vi "Select server and param_DO.vi"(0 "Activate":bool) -> (3 "This VI":refnum<vi>, 4 "host out":T1, 6 "HOST OK":bool, 12 "DI OK":bool, 13 "DI":string[](array[string]), 14 "DI table out":string="EP_XQ.1801" caption="таблица дискретных параметров")   [LabVIEW 2019]
uses:
  Database/PostgreSQL2LabVIEW/libpqlv/src/PQconnectdb.vi
  Database/PostgreSQL2LabVIEW/libpqlv/src/PQerrorMessage.vi
  Database/PostgreSQL2LabVIEW/libpqlv/src/PQstatus.vi
  Database/PostgreSQL2LabVIEW/libpqUtility/src/PQgetColumn.vi
  Database/PostgreSQL2LabVIEW/libpqUtility/src/PQclose.vi
  Database/select_initial.vi
  Database/PostgreSQL2LabVIEW/libpqlv/src/PQgetResult.vi
  Database/PostgreSQL2LabVIEW/libpqlv/src/PQclear.vi
  Database/PostgreSQL2LabVIEW/libpqUtility/src/PQfetchTables.vi
  Database/PostgreSQL2LabVIEW/libpqlv/src/PQresultErrorMessage.vi
  Database/PostgreSQL2LabVIEW/libpqlv/src/PQresultStatus.vi
  Database/PostgreSQL2LabVIEW/libpqlv/src/PQsendQuery.vi
  Database/PostgreSQL2LabVIEW/libpqlv/src/PQgetvalue.vi
  Database/PostgreSQL2LabVIEW/libpqlv/src/PQntuples.vi
  Database/PostgreSQL2LabVIEW/libpqUtility/src/PQgetTable.vi
  Database/Progress.vi
  Database/PostgreSQL2LabVIEW/libpqUtility/libpqutility.lvlib
  Database/PostgreSQL2LabVIEW/libpqlv/libpqlv.lvlib
  Inputs.lvlib
panel:
  in  "Param":i32[](listbox) caption="Параметры"
  in  "DI0":u16(ring) items=["EB31TB1_XB01", "EB31TB1_XB02", "EB31TB1_XB47", "EB321TB1_XB01", "EB321TB1_XB02", "EB321TB1_XB47", "EB322TB1_XB01", "EB322TB1_XB02", "EB322TB1_XB47", "EB323TB1_XB01", "EB323TB1_XB02", "EB323TB1_XB47", "EPCL1QM1_XB01", "EPCL1QM1_XB02", "EPCL1QM1_XB24", "EPG1GP1_XB01", "EPG1GP1_XB02", "EPG1GP1_XB19", "EPG1GP1_XB24", "EPG1GP2_XB01", "EPG1GP2_XB02", "EPG1GP2_XB19", "EPG1GP2_XB24", "EPG2GP1_XB01", "EPG2GP1_XB02", "EPG2GP1_XB19", "EPG2GP1_XB24", "EPG2GP2_XB01", "EPG2GP2_XB02", "EPG2GP2_XB19", "EPG2GP2_XB24", "EPG2GP3_XB01", "EPG2GP3_XB02", "EPG2GP3_XB19", "EPG2GP3_XB24", "EPG3GP1_XB01", "EPG3GP1_XB02", "EPG3GP1_XB19", "EPG3GP1_XB24", "EPG3GP2_XB01", "EPG3GP2_XB02", "EPG3GP2_XB19", "EPG3GP2_XB24", "EPHQ_XB01", "EPHQ_XB24", "EPKF1_A11", "EPKF1_A12", "EPKF1_A13", "EPKF1_A14", "EPKF1_A15", "EPKF2_A1", "EPKF2_A2", "EPKF2_A3", "GM31QM3_XB01", "GM31QM3_YB01", "GM31QM4_XB01", "GM31QM4_YB01", "HXQM1_XB01", "HXQM2_XB01", "HXQM3_XB01", "HXQM4_XB01", "HXQM5_XB01", "W1QM1_XB01", "W1QM1_YB01", "W1QM21_XB01", "W1QM21_YB01", "W1QM22_XB01", "W1QM22_YB01", "W1QM2_XB01", "W1QM2_YB01", "W1QM311_XB01", "W1QM311_YB01", "W1QM312_XB01", "W1QM312_YB01", "W1QM31_XB01", "W1QM31_YB01", "W1QM32_XB01", "W1QM32_YB01", "W1QM33_XB01", "W1QM33_YB01", "W1QM34_XB01", "W1QM34_YB01", "W1QM35_XB01", "W1QM35_YB01", "W1QM4_XB01", "W1QM4_YB01", "W1QM5_XB01", "W1QM5_YB01"]
  in  "DIParameters table":dbl[][](array[numeric])=[[0.0, 0.0, 3.0, 0.0], [0.0, 0.0, 3.0, 1.0], [0.0, 0.0, 0.0, 0.0], [0.0, 0.0, 3.0, 2.0], [0.0, 0.0, 3.0, 3.0], [0.0, 0.0, 3.0, 4.0], [0.0, 0.0, 0.0, 1.0], [0.0, 0.0, 3.0, 5.0], [0.0, 0.0, 4.0, 0.0], [0.0, 0.0, 4.0, 1.0], [0.0, 0.0, 0.0, 2.0], [0.0, 0.0, 4.0, 2.0], [0.0, 0.0, 4.0, 3.0], [0.0, 0.0, 4.0, 4.0], [0.0, 0.0, 0.0, 3.0], [0.0, 0.0, 4.0, 5.0], [0.0, 0.0, 4.0, 8.0], [0.0, 0.0, 4.0, 9.0], [0.0, 0.0, 0.0, 4.0], [0.0, 0.0, 4.0, 10.0], [0.0, 0.0, 7.0, 1.0], [0.0, 0.0, 7.0, 0.0], [0.0, 0.0, 0.0, 5.0], [0.0, 0.0, 7.0, 2.0], [0.0, 0.0, 7.0, 4.0], [0.0, 0.0, 7.0, 3.0], [0.0, 0.0, 0.0, 6.0], [0.0, 0.0, 7.0, 5.0], [0.0, 0.0, 3.0, 6.0], [0.0, 0.0, 3.0, 7.0], [0.0, 0.0, 4.0, 6.0], [0.0, 0.0, 0.0, 7.0], [0.0, 0.0, 4.0, 7.0], [0.0, 0.0, 0.0, 11.0], [0.0, 0.0, 0.0, 12.0], [0.0, 0.0, 0.0, 16.0], [0.0, 0.0, 0.0, 14.0], [0.0, 0.0, 0.0, 15.0], [0.0, 0.0, 0.0, 16.0], [0.0, 0.0, 0.0, 17.0], [0.0, 0.0, 0.0, 18.0]]
  in  "DINames":string[](array[string])=["Система охлаждения насосая станция циркуляции градирни 11 кВт насос 1 включен", "Система охлаждения насосая станция циркуляции градирни 11 кВт насос 1 отключен", "Система охлаждения насосая станция циркуляции градирни 11 кВт насос 1 есть питание", "Система охлаждения насосая станция циркуляции градирни 11 кВт насос 1 ручной", "Система охлаждения насосая станция циркуляции градирни 11 кВт насос 2 включен", "Система охлаждения насосая станция циркуляции градирни 11 кВт насос 2 отключен", "Система охлаждения насосая станция циркуляции градирни 11 кВт насос 2 есть питание", "Система охлаждения насосая станция циркуляции градирни 11 кВт насос 2 ручной", "Система охлаждения насосая станция циркуляции дистиллята насос 1 включен", "Система охлаждения насосая станция циркуляции дистиллята насос 1 отключен", "Система охлаждения насосая станция циркуляции дистиллята насос 1 есть питание", "Система охлаждения насосая станция циркуляции дистиллята насос 1 ручной", "Система охлаждения насосая станция циркуляции дистиллята насос 2 включен", "Система охлаждения насосая станция циркуляции дистиллята насос 2 отключен", "Система охлаждения насосая станция циркуляции дистиллята насос 2 есть питание", "Система охлаждения насосая станция циркуляции дистиллята насос 2 ручной", "Система охлаждения насосая станция циркуляции дистиллята насос агломератора включен", "Система охлаждения насосая станция циркуляции дистиллята насос агломератора отключен", "Система охлаждения насосая станция циркуляции дистиллята насос агломератора есть питание", "Система охлаждения насосая станция циркуляции дистиллята насос агломератора ручной", "Система охлаждения насосая станция циркуляции градирни 15 кВт насос 1 включен", "Система охлаждения насосая станция циркуляции градирни 15 кВт насос 1 отключен", "Система охлаждения насосая станция циркуляции градирни 15 кВт насос 1 есть питание", "Система охлаждения насосая станция циркуляции градирни 15 кВт насос 1 ручной", "Система охлаждения насосая станция циркуляции градирни 15 кВт насос 2 включен", "Система охлаждения насосая станция циркуляции градирни 15 кВт насос 2 отключен", "Система охлаждения насосая станция циркуляции градирни 15 кВт насос 2 есть питание", "Система охлаждения насосая станция циркуляции градирни 15 кВт насос 2 ручной", "Система охлаждения установка обратного осмоса включен", "Система охлаждения установка обратного осмоса ручной", "Система охлаждения емкость охлажденной воды клапан наполнения бака охлажденной воды включен", "Система охлаждения емкость охлажденной воды клапан наполнения бака охлажденной воды отключен", "Система охлаждения емкость охлажденной воды клапан наполнения бака охлажденной воды ручной", "Система охлаждения шкаф управления 1 есть связь", "Система охлаждения шкаф управления 1 есть связь", "Система охлаждения шкаф управления 1 есть связь", "Система охлаждения шкаф управления 1 есть связь", "Система охлаждения шкаф управления 1 есть связь", "Система охлаждения шкаф управления 2 есть связь", "Система охлаждения шкаф управления 2 есть связь", "Система охлаждения шкаф управления 2 есть связь"]
  in  "AIParameters table":dbl[][](array[numeric])=[[1.0, 0.0, 1000.0, 2.0, 0.0, 0.0, 1.0, 2.0, 6.0, 8.0, 100.0, 10.0, 2.0, 0.0, 6553.0, 32767.0, 0.0, 10.0, 1.0, 2.0, nan], [1.0, 0.0, 1000.0, 2.0, 0.0, 0.0, 1.0, 2.0, 6.0, 7.0, 100.0, 10.0, 2.0, 0.0, 6553.0, 32767.0, 0.0, 10.0, 1.0, 3.0, nan], [1.0, 0.0, 1000.0, 2.0, 0.0, 0.0, 1.0, 2.0, 6.0, 8.0, 10.0, 10.0, 2.0, 0.0, 6553.0, 32767.0, 0.0, 10.0, 2.0, 2.0, nan], [1.0, 0.0, 1000.0, 2.0, 0.0, 0.0, 1.0, 2.0, 6.0, 8.0, 10.0, 10.0, 2.0, 0.0, 6553.0, 32767.0, 0.0, 10.0, 2.0, 3.0, nan], [1.0, 0.0, 1000.0, 2.0, 0.0, 0.0, 3.0, 4.0, 7.0, 9.0, 10.0, 10.0, 2.0, 0.0, 6553.0, 32767.0, 0.0, 10.0, 2.0, 7.0, nan], [1.0, 0.0, 2000.0, 2.0, 0.0, 0.0, 1.0, 10.0, nan, 90.0, 100.0, 100.0, 2.0, 1.0, 6553.0, 32767.0, 0.0, 100.0, 1.0, 0.0, nan], [1.0, 0.0, 2000.0, 2.0, 0.0, 0.0, 1.0, 10.0, nan, 90.0, 100.0, 100.0, 2.0, 1.0, 6553.0, 32767.0, 0.0, 100.0, 1.0, 1.0, nan], [1.0, 0.0, 2000.0, 2.0, 0.0, 0.0, 1.0, 10.0, nan, 90.0, 100.0, 100.0, 2.0, 1.0, 6553.0, 32767.0, 0.0, 100.0, 2.0, 0.0, nan], [1.0, 0.0, 2000.0, 2.0, 0.0, 0.0, 1.0, 10.0, 60.0, 90.0, 100.0, 100.0, 2.0, 1.0, 6553.0, 32767.0, 0.0, 100.0, 2.0, 1.0, nan], [1.0, 0.0, 2000.0, 2.0, 0.0, 0.0, 40.0, 60.0, 120.0, nan, 250.0, 100.0, 2.0, 2.0, 6553.0, 32767.0, 0.0, 250.0, 1.0, 4.0, nan], [1.0, 0.0, 2000.0, 2.0, 0.0, 0.0, 30.0, 50.0, 150.0, nan, 250.0, 250.0, 2.0, 2.0, 6553.0, 32767.0, 0.0, 250.0, 2.0, 4.0, nan], [1.0, 0.0, 1000.0, 2.0, 0.0, 0.0, nan, 10.0, nan, nan, 100.0, 100.0, 2.0, 0.0, 6553.0, 32767.0, 0.0, 50.0, 1.0, 5.0, nan], [1.0, 0.0, 1000.0, 2.0, 0.0, 0.0, nan, 10.0, nan, nan, 100.0, 100.0, 2.0, 0.0, 6553.0, 32767.0, 0.0, 50.0, 1.0, 6.0, nan], [1.0, 0.0, 1000.0, 2.0, 0.0, 0.0, nan, 10.0, nan, nan, 50.0, 50.0, 2.0, 0.0, 6553.0, 32767.0, 0.0, 50.0, 2.0, 5.0, nan], [1.0, 0.0, 1000.0, 2.0, 0.0, 0.0, nan, 10.0, nan, nan, 50.0, 50.0, 2.0, 0.0, 6553.0, 32767.0, 0.0, 50.0, 2.0, 6.0, nan], [1.0, 0.0, 1000.0, 2.0, 0.0, 0.0, nan, 10.0, nan, nan, 50.0, 50.0, 2.0, 0.0, 6553.0, 32767.0, 0.0, 50.0, 6.0, 0.0, nan], [1.0, 0.0, 1000.0, 2.0, 0.0, 0.0, nan, 10.0, nan, nan, 50.0, 50.0, 2.0, 0.0, 6553.0, 32767.0, 0.0, 50.0, 6.0, 1.0, nan]] format="%#.3g"
  in  "AINames":string[][](array[string])=[["Система охлаждения давление охл. воды на входе в теплообменник", "bar"], ["Система охлаждения давление охлаждающей воды на выходе из теплообм", "bar"], ["Система охлаждения давление дистиллята на входе в теплообменник", "bar"], ["Система охлаждения давление дистиллята на входе в реактор", "bar"], ["Система охлаждения давление дистиллята на входе в агломератор", "bar"], ["Система охлаждения темпер. охлаждающей воды на входе в теплообменник", "oC"], ["Система охлаждения темп. охлаждающей воды на выходе из теплообменника", "oC"], ["Система охлаждения температура дистиллята на входе в теплообменник", "oC"], ["Система охлаждения температура дистиллята на выходе из теплообменника", "oC"], ["Система охлаждения емкость охлажденной воды уровень воды в емкости охлажденной воды", "mm"], ["Система охлаждения емкость дистиллята уровень в емкости дистиллята", "mm"], ["Система охлаждения насосая станция циркуляции градирни 11 кВт насос 1 контроль частоты", "Hz"], ["Система охлаждения насосая станция циркуляции градирни 11 кВт насос 2 контроль частоты", "Hz"], ["Система охлаждения насосая станция циркуляции дистиллята насос 1 контроль частоты", "Hz"], ["Система охлаждения насосая станция циркуляции дистиллята насос 2 контроль частоты", "Hz"], ["Система охлаждения насосая станция циркуляции градирни 15 кВт насос 1 контроль частоты", "Hz"], ["Система охлаждения насосая станция циркуляции градирни 15 кВт насос 2 контроль частоты", "Hz"]]
  in  "OK":bool
  in  "DI OK curr":bool
  in  "HOST OK curr":bool
  out "status":string="нет соединения" caption="состояние"
  in  "connect":bool
  in  "DI table":string="AZ1_XB" caption="таблица дискретных параметров"
  in  "host":string="192.168.36.191" caption="сервер"
  in  "password":string="Pht3833449525" caption="пароль"
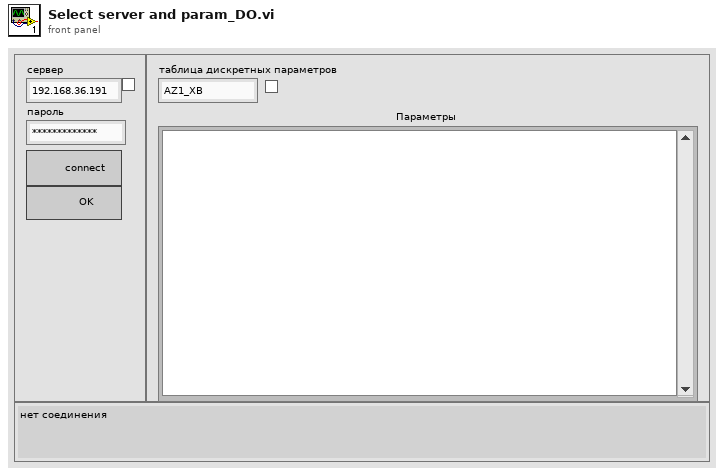
[diagram p1: front panel]
types:
  T1 = cluster{"host":string, "port":string, "client_encoding":string, "dbname":string, "user":string, "password":string}
  T2 = enum32{"CONNECTION_OK", "CONNECTION_BAD", "CONNECTION_STARTED", "CONNECTION_MADE", "CONNECTION_AWAITING_RESPONSE", "CONNECTION_AUTH_OK", "CONNECTION_SETENV", "CONNECTION_SSL_STARTUP", "CONNECTION_NEEDED"}
  T3 = enum32{"Invalid", "Standard", "Closed", "Hidden", "Minimized", "Maximized"}
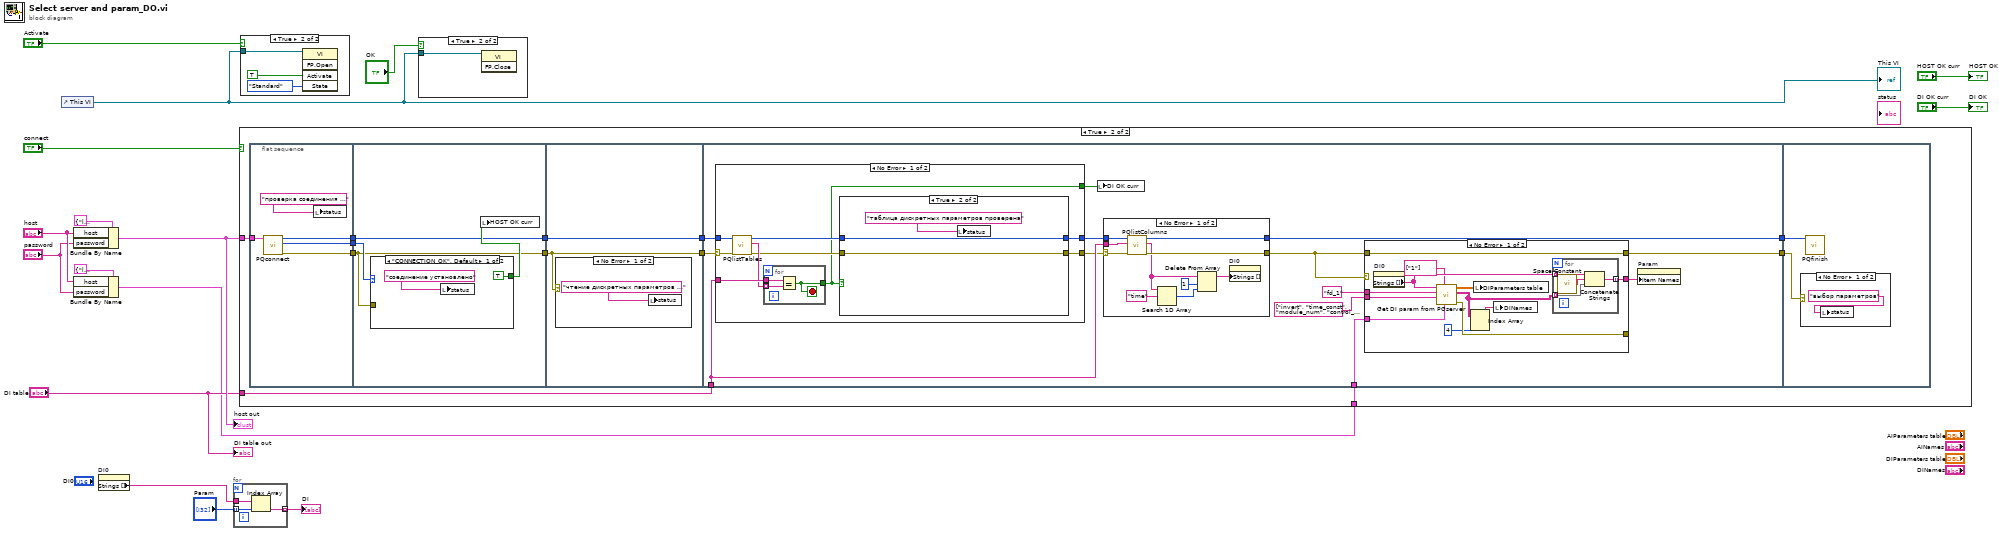
[diagram p0: block diagram]
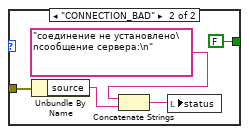
[diagram p3: hidden frame]
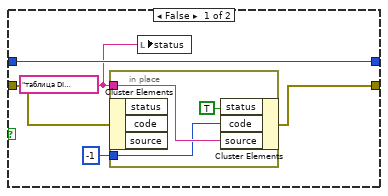
[diagram p6: hidden frame]
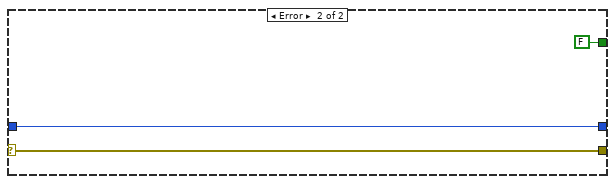
[diagram p7: hidden frame]
diagram:
  n1 = control-ref of="This VI"() -> (w9:refnum<vi>)
  "This VI" <- w9
  n2 = Bundle By Name(cluster=T1 {"host"="localhost", "port"="5432", "client_encoding"="LATIN1", "dbname"="data", "user"="postgres", "password"="ghjvfdnj1115"} ("conninfo"), "host"="host", "password"="password") -> (w15:T1)
  "host out" <- w15
  n3 = Bundle By Name(cluster=T1 {"host"="localhost", "port"="5432", "client_encoding"="LATIN1", "dbname"="system", "user"="postgres", "password"="ghjvfdnj1115"} ("conninfo"), "host"="host", "password"="password") -> (w4:T1)
  n4 = property on="DI0" class="Ring (strict)"() -> ("Strings []"=w3:string[])  [unwired: 2 in, 2 out]
  n5 = for {
    tunnel: w3 -> [w19]
    tunnel: "Param" -> [w17] mode=indexing
    tunnel: [w18] -> w1 mode=indexing
    n6 = Index Array(array=w19, index=w17) -> (element=w18:string)
  }
  "DI" <- w1
  n7 = case shown="True" "connect" {
    tunnel: w15 -> [_ w26]
    tunnel: "DI table" -> [_ w25]
    tunnel: w4 -> [_ w22]
    frame False {
    }
    frame True {
      n8 = flat-sequence {
        tunnel: w26 -> [w34]
        tunnel: [w36] -> w31
        tunnel: [w35] -> w30
        tunnel: [w33] -> w29
        tunnel: w31 -> [w38]
        tunnel: w30 -> [w37]
        tunnel: w29 -> [w40]
        tunnel: [w38] -> w21
        tunnel: [w37] -> w20
        tunnel: [w49] -> w28
        tunnel: [w48] -> w27
        tunnel: w21 -> [w49]
        tunnel: w20 -> [w48]
        tunnel: w28 -> [w63]
        tunnel: w27 -> [w62]
        tunnel: w25 -> [w61]
        tunnel: [w58] -> w24
        tunnel: [w53] -> w23
        tunnel: w22 -> [w52]
        tunnel: w24 -> [w119]
        tunnel: w23 -> [w120]
        frame #0 {
          n9 = call "PQconnect.vi"("conninfo"=w34) -> ("error out"=w35:errorcluster, "PQStatus"=w33:T2, "conn"=w36:u32)  [unwired: 8 in]
          n10 = local write "status"("проверка соединения ..." ("status")) -> ()
        }
        frame #1 {
          n11 = case shown="\"CONNECTION_OK\", Default" w40 {
            tunnel: w37 -> [_ w47]
            tunnel: [TRUE FALSE] -> w39
            frame "CONNECTION_OK", Default {
              n12 = local write "status"("соединение установлено" ("status")) -> ()
            }
            frame "CONNECTION_BAD" {
              n13 = Unbundle By Name(w47) -> ("source"=w46:string)
              n14 = Concatenate Strings("соединение не установлено\nсообщение сервера:\n" ("status"), w46) -> (w44:string)
              n15 = local write "status"(w44) -> ()
            }
          }
          n16 = local write "HOST OK curr"(w39) -> ()
        }
        frame #2 {
          n17 = case shown="No Error" w48 {
            frame No Error {
              n18 = local write "status"("чтение дискретных параметров ..." ("status")) -> ()
            }
            frame Error {
            }
          }
        }
        frame #3 {
          n19 = case shown="No Error" w62 {
            selector: w62 -> [w80 w101]
            tunnel: w63 -> [w81 w100]
            tunnel: [w84 w100] -> w60
            tunnel: [w83 w101] -> w59
            tunnel: w61 -> [w82 _]
            tunnel: [w76 FALSE] -> w57
            frame No Error {
              n20 = call "PQlistTables.vi"("error in"=w80, "conn"=w81) -> ("error out"=w77:errorcluster, "Data"=w79:string[], "conn_out"=w78:u32)  [unwired: 7 in]
              n21 = for {
                tunnel: w79 -> [w86] mode=indexing
                tunnel: w82 -> [w87]
                tunnel: [w85] -> w76
                stop <- w85 stop-if-true
                n22 = Equal?(x=w87, y=w86) -> (x = y?=w85:bool)
              }
              n23 = case shown="True" w76 {
                tunnel: w78 -> [w89 w98]
                tunnel: [w89 w98] -> w84
                tunnel: w77 -> [w90 w97]
                tunnel: [w91 w97] -> w83
                frame False {
                  w88 = "таблица DI отсутствует" ("source")
                  n24 = in-place {
                    in-place-border: w88 -> [w95]
                    in-place-border: -1 ("code") -> [w93]
                    n25 = in-place-cluster #1(w90) -> ()  [unwired: 3 out]
                    n26 = in-place-cluster #1("status"=TRUE, "code"=w93, "source"=w95) -> (w91:errorcluster)
                  }
                  n27 = local write "status"(w88) -> ()
                }
                frame True {
                  n28 = local write "status"("таблица дискретных параметров проверена" ("status")) -> ()
                }
              }
            }
            frame Error {
            }
          }
          n29 = local write "DI OK curr"(w57) -> ()
          n30 = case shown="No Error" w59 {
            selector: w59 -> [w71 w75]
            tunnel: [w69 w75] -> w54
            tunnel: [w72 w74] -> w58
            tunnel: w60 -> [w73 w74]
            tunnel: w61 -> [w70 _]
            frame No Error {
              n31 = call "PQlistColumns.vi"("error in"=w71, "table"=w70, "conn"=w73) -> ("error out"=w69:errorcluster, "Data"=w67:string[], "conn_out"=w72:u32)  [unwired: 6 in]
              n32 = Search 1D Array(1D array=w67, element="time") -> (index of element=w65:i32)  [unwired: 1 in]
              n33 = Delete From Array(array=w67, length=1, index=w65) -> (array with subset deleted=w64:string[])  [unwired: 1 out]
              n34 = property on="DI0" class="Ring (strict)"("Strings []"=w64) -> ()  [unwired: 2 in, 2 out]
            }
            frame Error {
            }
          }
          n35 = case shown="No Error" w54 {
            tunnel: w52 -> [w111 _]
            tunnel: [w110 _] -> _
            tunnel: "fd_1" ("DIParamTable") -> [w113 _]
            tunnel: string[] ["invert", "time_const", "module_num", "control_channel_num", "fname"] ("DIParamColumns") -> [w112 _]
            tunnel: w54 -> [w108 w118]
            tunnel: [w108 w118] -> w53
            tunnel: [w106 _] -> w51
            frame No Error {
              n36 = property on="DI0" class="Ring (strict)"() -> ("Strings []"=w107:string[])  [unwired: 2 in, 2 out]
              n37 = call "Get DI param from PGserver.vi"("conninfo"=w111, "KFM"=string[] ["1"], "DIParamColumns"=w112, "DIParamTable"=w113, "DI_fcode_full"=w107) -> ("error out"=w110:errorcluster, "Names table"=w104:string[][], "DIParameters table"=w109:dbl[][])  [unwired: 4 in]
              n38 = Index Array(array=w104, index (col)=4 ("index (row)")) -> (element=w102:string[])  [unwired: 1 in]
              n39 = local write "DIParameters table"(w109) -> ()
              n40 = local write "DINames"(w102) -> ()
              n41 = for {
                tunnel: w107 -> [w117] mode=indexing
                tunnel: w104 -> [w115] mode=indexing
                tunnel: [w114] -> w106 mode=indexing
                n42 = call <vilib>:"Space Constant.vi"() -> ("String"=w116:string)
                n43 = Concatenate Strings(w117, w116, w115) -> (w114:string)
              }
            }
            frame Error {
            }
          }
          n44 = property on="Param" class="LstBox (strict)"("Item Names"=w51) -> ()  [unwired: 2 in, 2 out]
        }
        frame #4 {
          n45 = case shown="No Error" w120 {
            frame No Error {
              n46 = local write "status"("выбор параметров" ("status")) -> ()
            }
            frame Error {
            }
          }
          n47 = call "PQfinish.vi"("conn"=w119) -> ()  [unwired: 10 in, 1 out]
        }
      }
    }
  }
  n48 = case shown="True" "Activate" {
    tunnel: w9 -> [_ w123]
    frame False {
    }
    frame True {
      n49 = invoke class="VI" method="FP.Open"(reference=w123, "Activate"=TRUE ("Activate?"), "State"=T3."Standard") -> ()  [unwired: 2 in, 5 out]
    }
  }
  n50 = case shown="True" "OK" {
    tunnel: w9 -> [_ w125]
    frame False {
    }
    frame True {
      n51 = invoke class="VI" method="FP.Close"(reference=w125) -> ()  [unwired: 2 in, 3 out]
    }
  }
  "DI table out" <- "DI table"
  "HOST OK" <- "HOST OK curr"
  "DI OK" <- "DI OK curr"
